vi "SortClicks.vi"(7 "Table History ref":refnum<vi>, 8 "error in (no error)":errorcluster, 10 "ClickEvent in":T3, 11 "Col array in":refnum<class "Column.lvclass">[](array[class])) -> (0 "error out":errorcluster, 1 "Row Type":T2, 2 "Click out":T1, 3 "Col array out":refnum<class "Column.lvclass">[](array[class]), 4 "Update HWI?":bool, 5 "withinData?":bool=TRUE)   [LabVIEW 2013]
doc: "Specialize click-sorting for SetList Table. The case structure was forcing the Table control event loop within the main SetList program to be very large, so I've moved the click-sorting within this SubVI.\n\nFor an overview of how clicks are sorted, see the additional documentation (or read comments)."
uses:
  TypeDefs/ClickEvent.ctl
  <vilib>/Utility/miscctls.llb/LVPoint32TypeDef.ctl
  TypeDefs/TableHistory.ctl
  TypeDefs/TableArray.ctl
  ColumnVIs/Column/Column.lvclass
  TypeDefs/RowType.ctl
  TypeDefs/ClickReturn.ctl
  <vilib>/Utility/miscctls.llb/LVRowAndColumnTypeDef.ctl
  Globals/DisabledColorGlobal.vi
panel:
  out "disabled?":bool
  # "Change this typedef if LabVIEW changes what is provided on click event!"
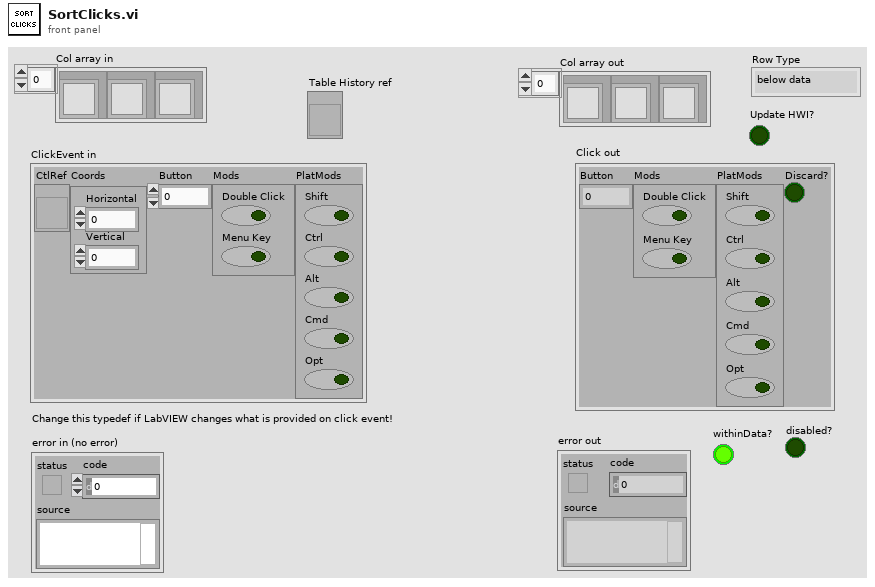
[diagram p1: front panel]
types:
  T1 = typedef "ClickReturn.ctl" = cluster{"Button":u16, "Mods":cluster{"Double Click":bool, "Menu Key":bool}, "PlatMods":cluster{"Shift":bool, "Ctrl":bool, "Alt":bool, "Cmd":bool, "Opt":bool}, "Discard?":bool}
  T2 = typedef "RowType.ctl" = enum16{"below data", "within data", "column header", "first row"}
  T3 = typedef "ClickEvent.ctl" = cluster{"CtlRef":refnum<vi>, "Coords":T4, "Button":u16, "Mods":cluster{"Double Click":bool, "Menu Key":bool}, "PlatMods":cluster{"Shift":bool, "Ctrl":bool, "Alt":bool, "Cmd":bool, "Opt":bool}}
  T4 = typedef "LVPoint32TypeDef.ctl" = cluster{"Horizontal":i32, "Vertical":i32}
  T5 = cluster{"Shift":bool, "Ctrl":bool, "Alt":bool, "Cmd":bool, "Opt":bool}
  T6 = typedef "LVRowAndColumnTypeDef.ctl" = cluster{"Row":i32, "Column":i32}
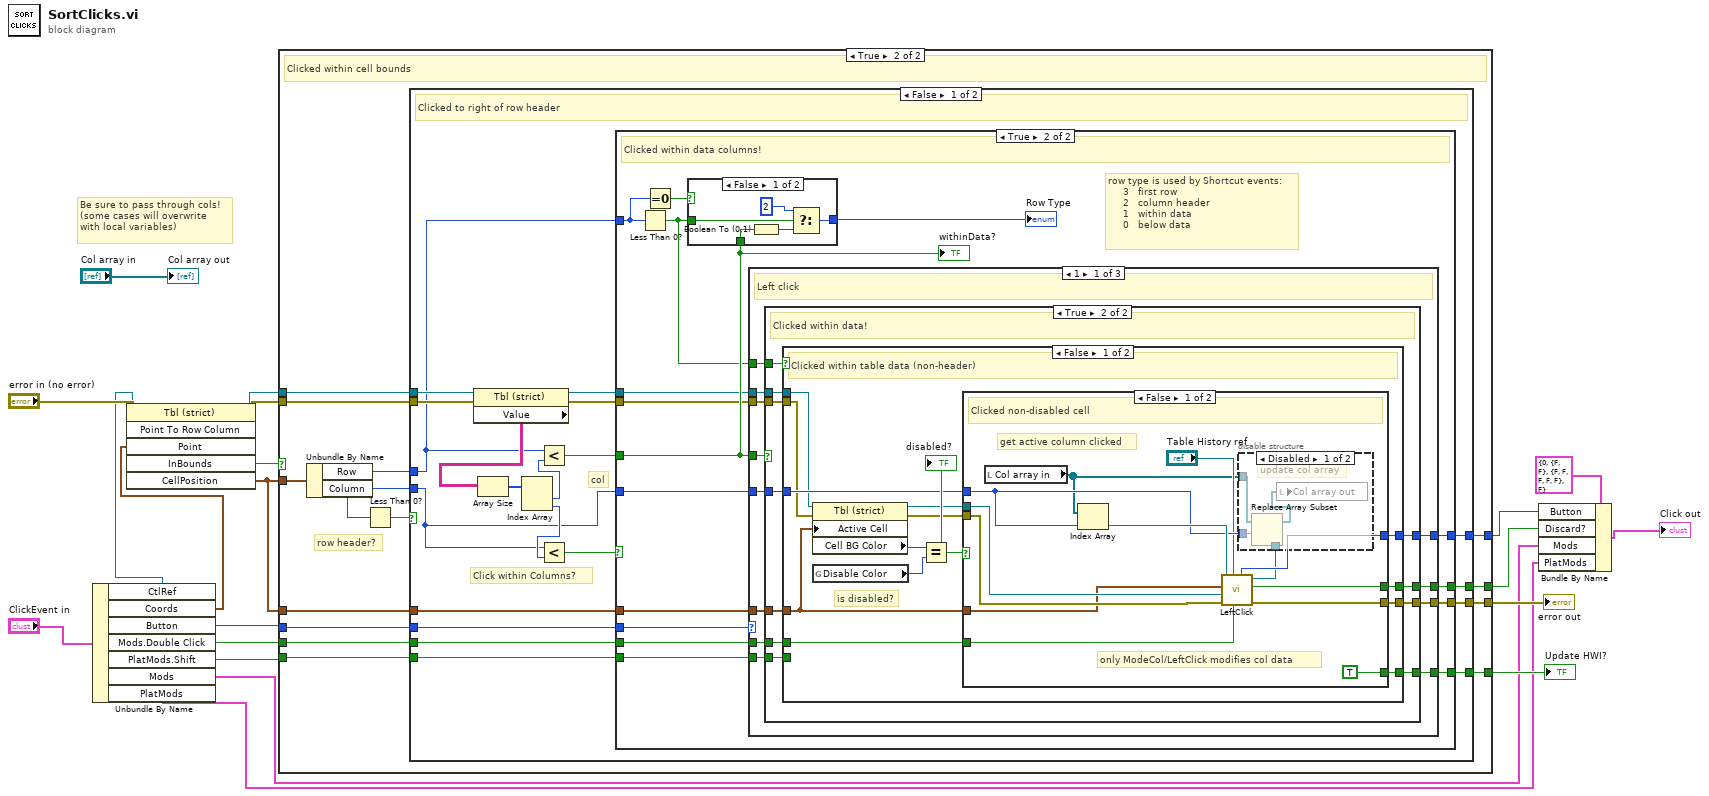
[diagram p0: block diagram]
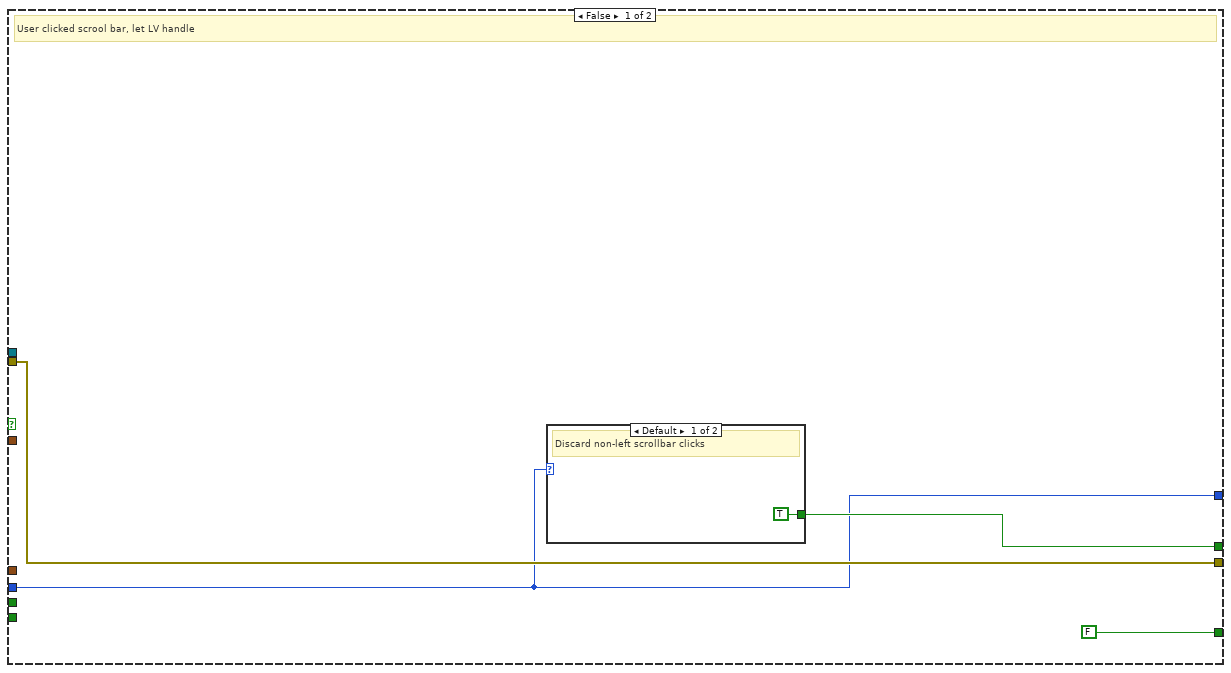
[diagram p2: hidden frame]
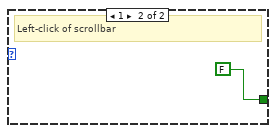
[diagram p3: hidden frame]
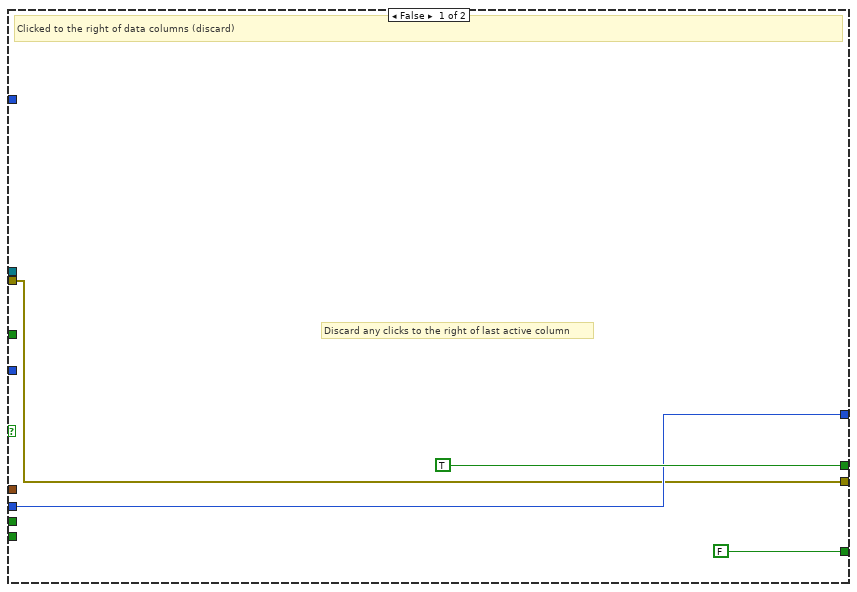
[diagram p4: hidden frame]
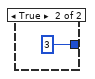
[diagram p5: hidden frame]
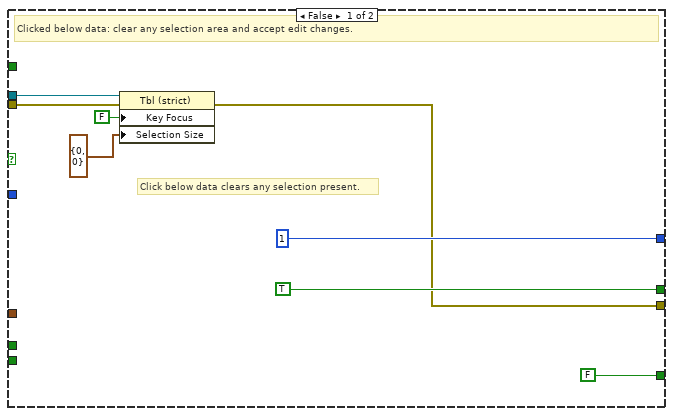
[diagram p6: hidden frame]
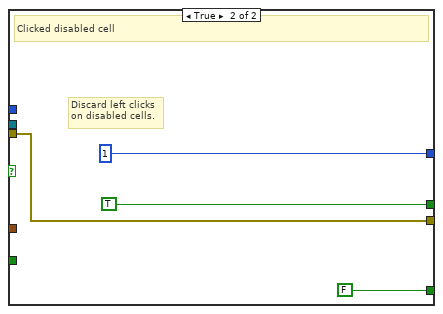
[diagram p8: hidden frame]
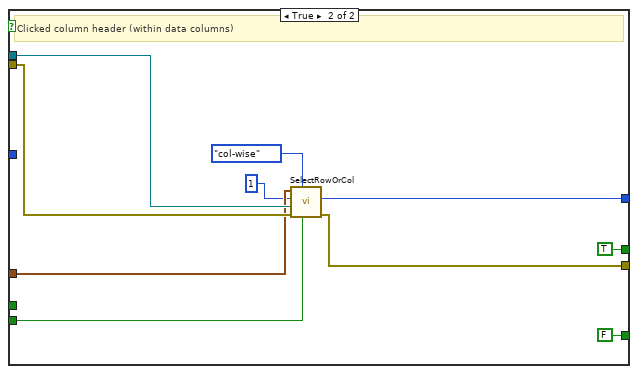
[diagram p9: hidden frame]
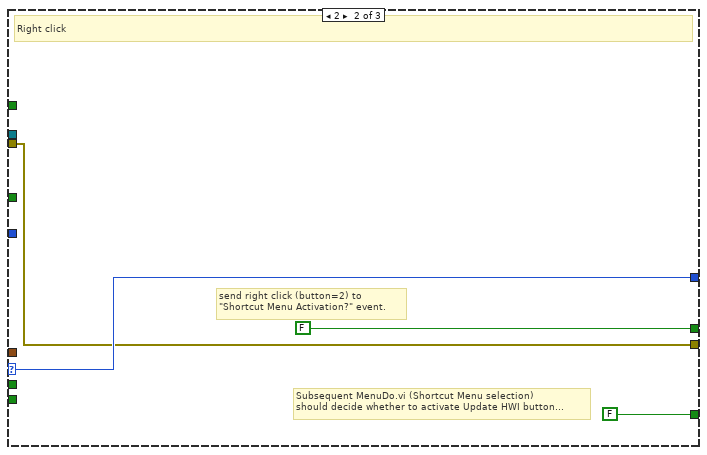
[diagram p10: hidden frame]
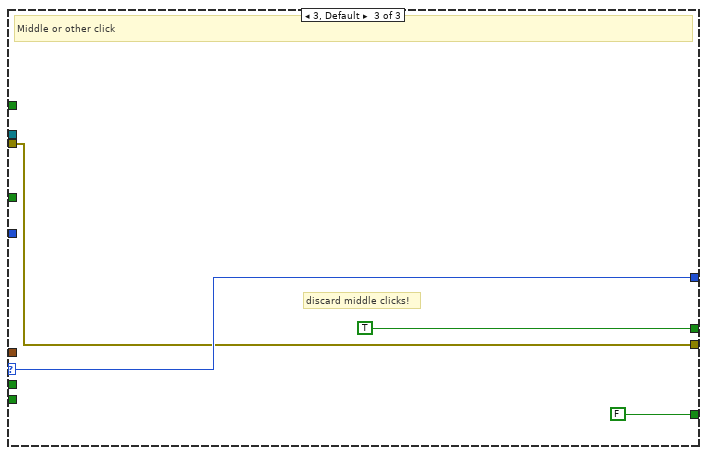
[diagram p11: hidden frame]
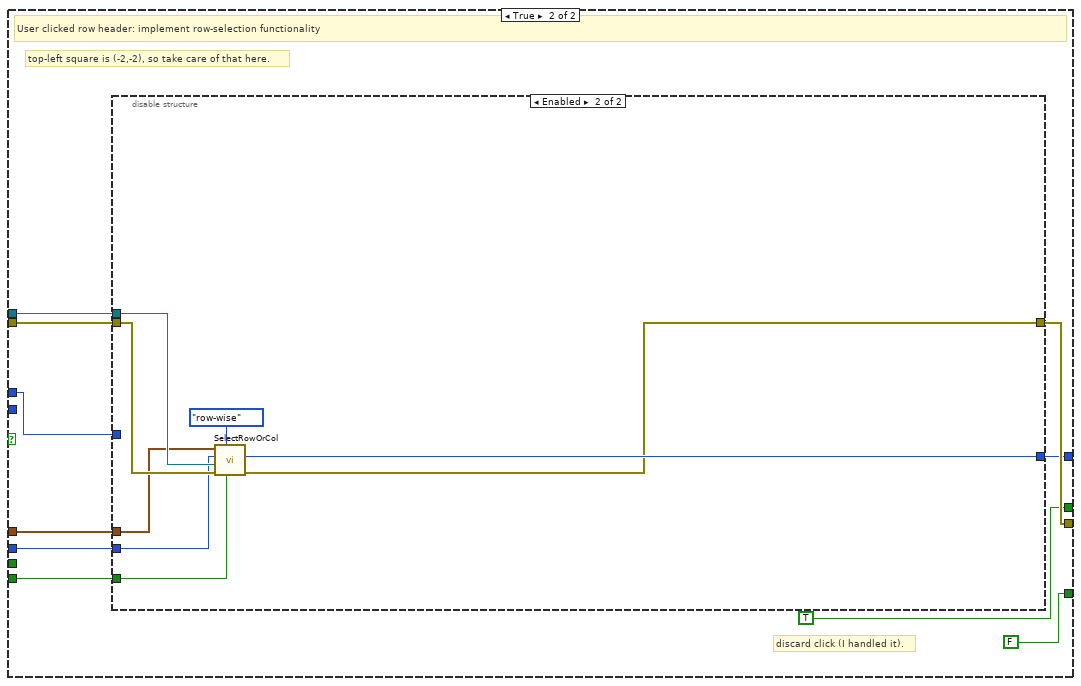
[diagram p12: hidden frame]
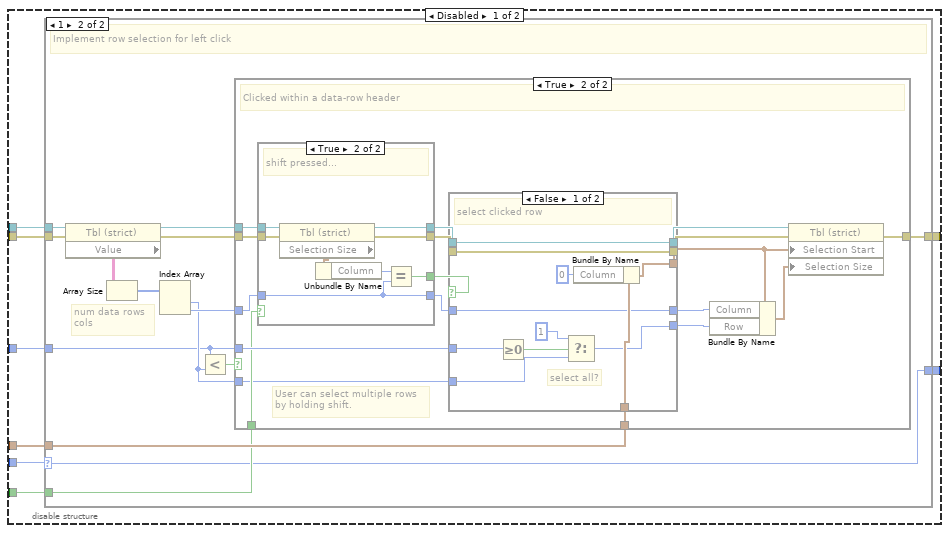
[diagram p13: hidden frame]
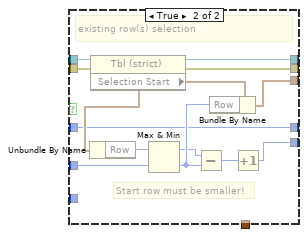
[diagram p16: hidden frame]
diagram:
  # "Be sure to pass through cols!\n(some cases will overwrite \nwith local variables)"
  n1 = Unbundle By Name("ClickEvent in") -> ("CtlRef"=w15:refnum<vi>, "Coords"=w11:T4, "Button"=w12:u16, "Mods.Double Click"=w14:bool, "PlatMods.Shift"=w13:bool, "Mods"=w2:cluster{"Double Click":bool, "Menu Key":bool}, "PlatMods"=w1:T5)
  n2 = invoke class="Tbl (strict)" method="Point To Row Column"(reference=w15, error in="error in (no error)", "Point"=w11) -> (reference out=w20:refnum<vi>, error out=w19:errorcluster, "InBounds"=w18:bool, "CellPosition"=w5:T6)  [unwired: 3 in, 2 out]
  n3 = case shown="True" w18 {
    tunnel: [w24 w38] -> w3
    tunnel: w5 -> [_ w40]
    tunnel: w19 -> [w23 w37]
    tunnel: w20 -> [_ w36]
    tunnel: w12 -> [w21 w33]
    tunnel: w14 -> [_ w30]
    tunnel: w5 -> [_ w31]
    tunnel: [w23 w29] -> w10
    tunnel: [w21 w32] -> w7
    tunnel: w13 -> [_ w28]
    tunnel: [FALSE w27] -> w6
    frame False {
      # "User clicked scrool bar, let LV handle"
      n4 = case shown="Default" w21 {
        tunnel: [TRUE FALSE] -> w24
        frame Default {
          # "Discard non-left scrollbar clicks"
        }
        frame 1 {
          # "Left-click of scrollbar"
        }
      }
    }
    frame True {
      # "row header?"
      # "Clicked within cell bounds"
      n5 = Unbundle By Name(w40) -> ("Row"=w35:i32, "Column"=w34:i32)
      n6 = Less Than 0?(x=w34) -> (x < 0?=w39:bool)
      n7 = case shown="False" w39 {
        tunnel: [w52 TRUE] -> w38
        tunnel: w35 -> [w42 w177]
        tunnel: w37 -> [w55 w179]
        tunnel: w36 -> [w56 w178]
        tunnel: w34 -> [w45 _]
        tunnel: w33 -> [w53 w174]
        tunnel: [w50 w172] -> w32
        tunnel: w31 -> [w47 w176]
        tunnel: w30 -> [w46 _]
        tunnel: [w44 w180] -> w29
        tunnel: w28 -> [w41 w175]
        tunnel: [w43 FALSE] -> w27
        frame False {
          # "col"
          # "Click within Columns?"
          # "Clicked to right of row header"
          n8 = property class="Tbl (strict)"(reference=w56, error in=w55) -> (reference out=w49:refnum<vi>, error out=w48:errorcluster, "Value"=w60:string[][])
          n9 = Array Size(array=w60) -> (size(s)=w59:i32[])
          n10 = Index Array(array=w59) -> (element #1=w58:i32, element #2=w57:i32)  [unwired: 2 in]
          n11 = Less?(x=w42, y=w58) -> (x < y?=w51:bool)
          n12 = Less?(x=w45, y=w57) -> (x < y?=w54:bool)
          n13 = case shown="True" w54 {
            tunnel: w51 -> [_ w74]
            tunnel: w53 -> [w63 w80]
            tunnel: [TRUE w79] -> w52
            tunnel: [w63 w78] -> w50
            tunnel: w49 -> [_ w72]
            tunnel: w48 -> [w62 w71]
            tunnel: w47 -> [_ w73]
            tunnel: w46 -> [_ w77]
            tunnel: w45 -> [_ w76]
            tunnel: [w62 w75] -> w44
            tunnel: w42 -> [_ w67]
            tunnel: [FALSE w68] -> w43
            tunnel: w41 -> [_ w65]
            frame False {
              # "Discard any clicks to the right of last active column"
              # "Clicked to the right of data columns (discard)"
            }
            frame True {
              # "row type is used by Shortcut events:\n     3   first row\n     2   column header\n     1   within data\n     0   below data"
              # "Clicked within data columns!"
              n14 = Less Than 0?(x=w67) -> (x < 0?=w66:bool)
              n15 = Equal To 0?(x=w67) -> (x = 0?=w70:bool)
              n16 = case shown="False" w70 {
                tunnel: [w83 i16 3] -> w69
                tunnel: w74 -> [w82 _]
                tunnel: w66 -> [w81 _]
                frame False {
                  n17 = Boolean To (0,1)(Boolean=w82) -> (0, 1=w84:i16)
                  n18 = Select(t=i16 2, s=w81, f=w84) -> (s? t:f=w83:i16)
                }
                frame True {
                }
              }
              "Row Type" <- w69
              n19 = case shown="1" w80 {
                selector: w80 -> [_ w165 w169]
                tunnel: [w97 FALSE TRUE ("Discard?")] -> w79
                tunnel: w74 -> [w98 _ _]
                tunnel: [w96 w165 w169] -> w78
                tunnel: w73 -> [w95 _ _]
                tunnel: w77 -> [w94 _ _]
                tunnel: w76 -> [w93 _ _]
                tunnel: [w92 w164 w168] -> w75
                tunnel: w72 -> [w91 _ _]
                tunnel: w71 -> [w90 w164 w168]
                tunnel: [w89 FALSE FALSE] -> w68
                tunnel: w66 -> [w88 _ _]
                tunnel: w65 -> [w87 _ _]
                frame 1 {
                  # "Left click"
                  n20 = case shown="True" w98 {
                    tunnel: [TRUE w117] -> w97
                    tunnel: [u16 1 w116] -> w96
                    tunnel: w95 -> [_ w112]
                    tunnel: w94 -> [_ w115]
                    tunnel: w93 -> [_ w114]
                    tunnel: [w101 w113] -> w92
                    tunnel: w91 -> [w103 w111]
                    tunnel: w90 -> [w102 w110]
                    tunnel: [FALSE w109] -> w89
                    tunnel: w88 -> [_ w108]
                    tunnel: w87 -> [_ w107]
                    frame False {
                      # "Click below data clears any selection present."
                      # "Clicked below data: clear any selection area and accept edit changes."
                      n21 = property class="Tbl (strict)"(reference=w103, error in=w102, "Key Focus"=FALSE, "Selection Size"=T6 {"Row"=0, "Column"=0}) -> (error out=w101:errorcluster)  [unwired: 1 out]
                    }
                    frame True {
                      # "Clicked within data!"
                      n22 = case shown="False" w108 {
                        tunnel: [w128 TRUE ("Discard?")] -> w117
                        tunnel: [w127 w153] -> w116
                        tunnel: w115 -> [w126 _]
                        tunnel: w114 -> [w125 _]
                        tunnel: [w122 w157] -> w113
                        tunnel: w112 -> [w121 w159]
                        tunnel: w111 -> [w120 w161]
                        tunnel: w110 -> [w119 w160]
                        tunnel: [w118 FALSE] -> w109
                        tunnel: w107 -> [_ w158]
                        frame False {
                          # "is disabled?"
                          # "Clicked within table data (non-header)"
                          n23 = property class="Tbl (strict)"(reference=w120, error in=w119, "Active Cell"=w121) -> (reference out=w124:refnum<vi>, error out=w123:errorcluster, "Cell BG Color"=w131:u32)
                          n24 = global read "DisabledColorGlobal.vi" "Disable Color"() -> (w130:u32)
                          n25 = Equal?(x=w131, y=w130) -> (x = y?=w129:bool)
                          "disabled?" <- w129
                          n26 = case shown="False" w129 {
                            tunnel: [w144 TRUE] -> w128
                            tunnel: [w141 u16 1] -> w127
                            tunnel: w126 -> [w135 _]
                            tunnel: w125 -> [w139 _]
                            tunnel: w124 -> [w138 _]
                            tunnel: w123 -> [w137 w150]
                            tunnel: [w142 w150] -> w122
                            tunnel: w121 -> [w136 _]
                            tunnel: [TRUE FALSE] -> w118
                            frame False {
                              # "only ModeCol/LeftClick modifies col data"
                              # "get active column clicked"
                              # "Clicked non-disabled cell"
                              n27 = local read "Col array in"() -> (w132:refnum<class "Column.lvclass">[])
                              n28 = Index Array(array=w132, index=w139) -> (element=w143:refnum<class "Column.lvclass">)
                              n29 = call-dynamic "LeftClick.vi"("Double Click"=w135, "Table History ref"="Table History ref", "error in (no error)"=w137, "Table CtlRef In"=w138, "Cell Position"=w136, "Column in"=w143) -> ("error out"=w142:errorcluster, "Discard?"=w144:bool, "Column out"=w140:refnum<class "Column.lvclass">, "Button"=w141:u16)  [unwired: 1 in, 1 out]
                              n30 = disable-structure shown="Disabled" {
                                disable-tunnel: w140 -> [w148 _]
                                disable-tunnel: w139 -> [w147 _]
                                disable-tunnel: w132 -> [w145 _]
                                frame Disabled {
                                # "update col array"
                                n31 = Replace Array Subset(array=w145, new element=w148, index=w147) -> (w146:refnum<class "Column.lvclass">[])
                                n32 = local write "Col array out"(w146) -> ()
                                }
                                frame Enabled {
                                }
                              }
                            }
                            frame True {
                              # "Discard left clicks\non disabled cells."
                              # "Clicked disabled cell"
                            }
                          }
                        }
                        frame True {
                          # "Clicked column header (within data columns)"
                          n33 = call "SelectRowOrCol.vi"("Shift Pressed? (F)"=w158, "Row/Col"=enum16{"row-wise", "col-wise"}."col-wise", "error in"=w160, "Table CtlRef"=w161, "Button (1)"=u16 1 ("Button"), "CellPosition"=w159) -> ("error out"=w157:errorcluster, "Button"=w153:u16)  [unwired: 4 in]
                        }
                      }
                    }
                  }
                }
                frame 2 {
                  # "Subsequent MenuDo.vi (Shortcut Menu selection)\nshould decide whether to activate Update HWI button..."
                  # "send right click (button=2) to \n\"Shortcut Menu Activation?\" event."
                  # "Right click"
                }
                frame 3, Default {
                  # "discard middle clicks!"
                  # "Middle or other click"
                }
              }
              "withinData?" <- w74
            }
          }
        }
        frame True {
          # "discard click (I handled it)."
          # "top-left square is (-2,-2), so take care of that here."
          # "User clicked row header: implement row-selection functionality"
          n34 = disable-structure shown="Enabled" {
            disable-tunnel: [w188 w263] -> w180
            disable-tunnel: w179 -> [w187 w266]
            disable-tunnel: w178 -> [w186 w267]
            disable-tunnel: w177 -> [w185 _]
            disable-tunnel: w176 -> [w184 w261]
            disable-tunnel: w175 -> [w183 w260]
            disable-tunnel: w174 -> [w182 w265]
            disable-tunnel: [w181 w264] -> w172
            frame Disabled {
              n35 = case shown="1" w182 {
                selector: w182 -> [w189 w195]
                tunnel: [w190 w204] -> w188
                tunnel: w187 -> [w190 w203]
                tunnel: w186 -> [_ w202]
                tunnel: w185 -> [_ w192]
                tunnel: w184 -> [_ w197]
                tunnel: w183 -> [_ w196]
                tunnel: [w189 w195] -> w181
                frame Default {
                }
                frame 1 {
                  # "num data rows\ncols"
                  # "Implement row selection for left click"
                  n36 = property class="Tbl (strict)"(reference=w202, error in=w203) -> (reference out=w199:refnum<vi>, error out=w198:errorcluster, "Value"=w201:string[][])
                  n37 = Array Size(array=w201) -> (size(s)=w200:i32[])
                  n38 = Index Array(array=w200) -> (element #1=w193:i32, element #2=w194:i32)  [unwired: 2 in]
                  n39 = Less?(x=w192, y=w193) -> (x < y?=w191:bool)
                  n40 = case shown="True" w191 {
                    tunnel: [w205 w223] -> w204
                    tunnel: w199 -> [_ w222]
                    tunnel: w198 -> [w205 w221]
                    tunnel: w192 -> [_ w215]
                    tunnel: w197 -> [_ w214]
                    tunnel: w196 -> [_ w208]
                    tunnel: w193 -> [_ w207]
                    tunnel: w194 -> [_ w206]
                    frame False {
                      # "ignore row clicks below data!"
                    }
                    frame True {
                      # "User can select multiple rows\nby holding shift."
                      # "Clicked within a data-row header"
                      n41 = case shown="True" w208 {
                        selector: w208 -> [w251 _]
                        tunnel: w222 -> [w250 w259]
                        tunnel: w221 -> [w249 w258]
                        tunnel: [w249 w257] -> w218
                        tunnel: [w250 w256] -> w220
                        tunnel: w206 -> [w248 w252]
                        tunnel: [w251 w253] -> w216
                        tunnel: [w248 w252] -> w213
                        frame False {
                        }
                        frame True {
                          # "shift pressed..."
                          n42 = property class="Tbl (strict)"(reference=w259, error in=w258) -> (reference out=w256:refnum<vi>, error out=w257:errorcluster, "Selection Size"=w255:T6)
                          n43 = Unbundle By Name(w255) -> ("Column"=w254:i32)
                          n44 = Equal?(x=w254, y=w252) -> (x = y?=w253:bool)
                        }
                      }
                      n45 = case shown="False" w216 {
                        tunnel: w220 -> [w234 w247]
                        tunnel: [w234 w246] -> w219
                        tunnel: w218 -> [w233 w245]
                        tunnel: [w233 w244] -> w217
                        tunnel: w215 -> [w228 w242]
                        tunnel: [w231 w241] -> w211
                        tunnel: w214 -> [w232 _]
                        tunnel: w213 -> [w229 w236]
                        tunnel: [w229 w236] -> w212
                        tunnel: [w226 w235] -> w209
                        tunnel: w207 -> [w224 _]
                        frame False {
                          # "select all?"
                          # "select clicked row"
                          n46 = Greater Or Equal To 0?(x=w228) -> (x >= 0?=w227:bool)
                          n47 = Select(t=1, s=w227, f=w224) -> (s? t:f=w226:i32)
                          n48 = Bundle By Name(cluster=w232, "Column"=0) -> (w231:T6)
                        }
                        frame True {
                          # "Start row must be smaller!"
                          # "existing row(s) selection"
                          n49 = property class="Tbl (strict)"(reference=w247, error in=w245) -> (reference out=w246:refnum<vi>, error out=w244:errorcluster, "Selection Start"=w237:T6)
                          n50 = Unbundle By Name(w237) -> ("Row"=w243:i32)
                          n51 = Max & Min(x=w243, y=w242) -> (max(x,y)=w239:i32, min(x,y)=w240:i32)
                          n52 = Subtract(x=w239, y=w240) -> (x-y=w238:i32)
                          n53 = Bundle By Name(cluster=w237, "Row"=w240) -> (w241:T6)
                          n54 = Increment(x=w238) -> (x+1=w235:i32)
                        }
                      }
                      n55 = Bundle By Name(cluster=w211, "Column"=w212, "Row"=w209) -> (w210:T6)
                      n56 = property class="Tbl (strict)"(reference=w219, error in=w217, "Selection Start"=w211, "Selection Size"=w210) -> (error out=w223:errorcluster)  [unwired: 1 out]
                    }
                  }
                }
              }
            }
            frame Enabled {
              n57 = call "SelectRowOrCol.vi"("Shift Pressed? (F)"=w260, "Row/Col"=enum16{"row-wise", "col-wise"}."row-wise", "error in"=w266, "Table CtlRef"=w267, "Button (1)"=w265, "CellPosition"=w261) -> ("error out"=w263:errorcluster, "Button"=w264:u16)  [unwired: 4 in]
            }
          }
        }
      }
    }
  }
  "error out" <- w10
  "Update HWI?" <- w6
  n58 = Bundle By Name(cluster=T1 {"Button"=0, "Mods"={"Double Click"=FALSE, "Menu Key"=FALSE}, "PlatMods"={"Shift"=FALSE, "Ctrl"=FALSE, "Alt"=FALSE, "Cmd"=FALSE, "Opt"=FALSE}, "Discard?"=FALSE} ("Click out"), "Button"=w7, "Discard?"=w3, "Mods"=w2, "PlatMods"=w1) -> (→"Click out":T1)
  "Col array out" <- "Col array in"
